vi "Decorate.vi"(10 "Actor":refnum<class "Actor.lvclass">, 11 "Base Actor in":refnum<class "Base Actor.lvclass">) -> (3 "Base Actor out":refnum<class "Base Actor.lvclass">)   [LabVIEW 2021, in "jettl.lvlib" / "Actor.lvlib" / "Base Actor.lvclass"]
uses:
  Base Actor.lvclass
  Actor/Actor.lvclass
  Base Actor.lvclass/Base Actor.ctl
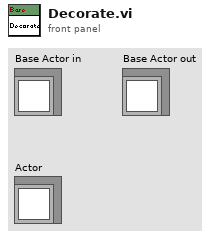
[diagram p1: front panel]
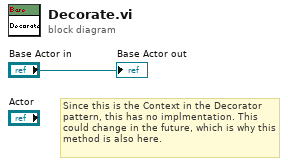
[diagram p0: block diagram]
diagram:
  # "Since this is the Context in the Decorator pattern, this has no implmentation. This could change in the future, which is why this method is also here."
  "Base Actor out" <- "Base Actor in"
